vi "GetFileList.vi"(8 "Error In":errorcluster caption="エラー入力", 10 "検索文字":string, 11 "フォルダパス":path) -> (0 "Error Out":errorcluster caption="エラー出力", 3 "ファイルリスト":string[](array[string]))   [LabVIEW 2014]
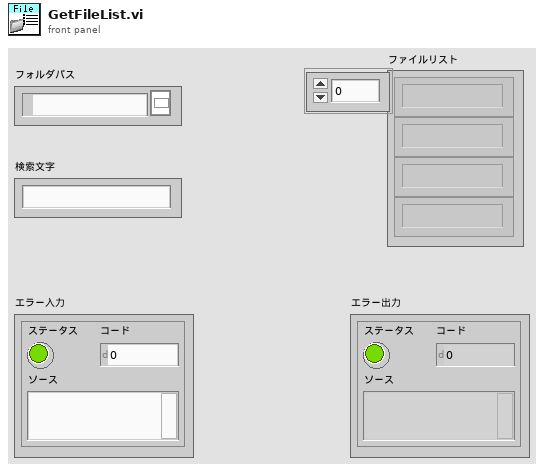
[diagram p1: front panel]
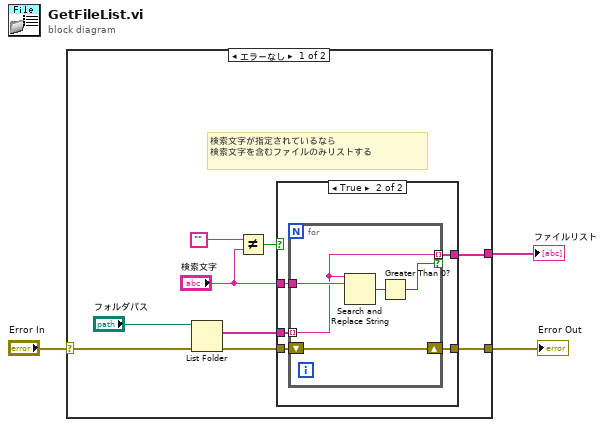
[diagram p0: block diagram]
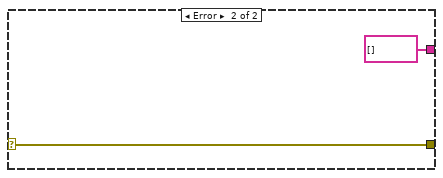
[diagram p3: hidden frame]
diagram:
  n1 = case shown="エラーなし" "Error In" {
    selector: "Error In" -> [w12 w26]
    tunnel: [w8 w26] -> w2
    tunnel: [w7 string[] []] -> w1
    frame No Error {
      # "検索文字が指定されているなら\n検索文字を含むファイルのみリストする"
      n2 = List Folder(path="フォルダパス", error in=w12) -> (filenames=w9:string[], error out=w10:errorcluster)  [unwired: 2 in, 2 out]
      n3 = Not Equal?(x="", y="検索文字") -> (x != y?=w4:bool)
      n4 = case shown="TRUE" w4 {
        tunnel: w10 -> [w13 w19]
        tunnel: w9 -> [w14 w18]
        tunnel: [w13 w17] -> w8
        tunnel: [w14 w16] -> w7
        tunnel: "検索文字" -> [_ w15]
        frame False {
        }
        frame True {
          n5 = for {
            shift-right: [w24] -> w17
            shift-left: w19 -> [w24]
            tunnel: w18 -> [w22] mode=indexing
            tunnel: w15 -> [w23]
            tunnel: [w22] -> w16 mode=indexing if=w20
            n6 = Search and Replace String(input string=w22, search string=w23) -> (number of replacements=w21:i32)  [unwired: 6 in, 3 out]
            n7 = Greater Than 0?(x=w21) -> (x > 0?=w20:bool)
          }
        }
      }
    }
    frame Error {
    }
  }
  "Error Out" <- w2
  "ファイルリスト" <- w1
